vi "Write Size.vi"(8 "error in (no error)":errorcluster, 10 "Coordinate":T1, 11 "Menu in":refnum<class "Menu.lvclass">) -> (0 "error out":errorcluster, 3 "Menu out":refnum<class "Menu.lvclass">)   [LabVIEW 2019, in "RT_Game.lvlib" / "Menu.lvclass"]
uses:
  Menu.lvclass
  Game/Coordinate.ctl
  Menu.lvclass/Menu.ctl
  Game/Game.lvclass
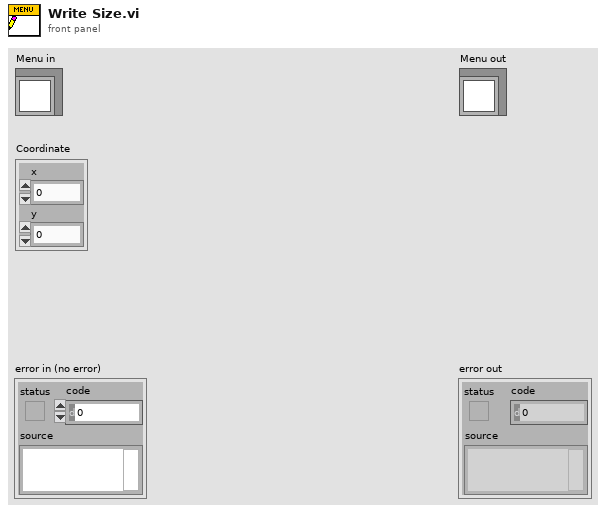
[diagram p1: front panel]
types:
  T1 = typedef "RT_Game.lvlib/Game.lvclass/Coordinate.ctl" = cluster{"x":i16, "y":i16}
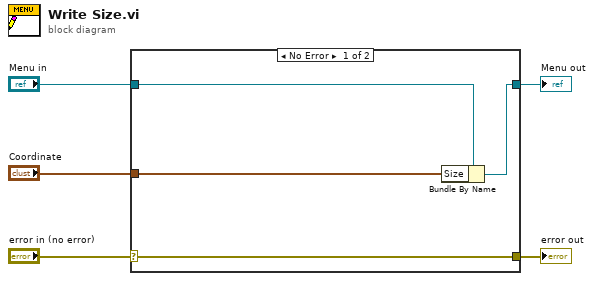
[diagram p0: block diagram]
diagram:
  n1 = case shown="No Error" "error in (no error)" {
    selector: "error in (no error)" -> [w9 w10]
    tunnel: [w9 w10] -> w4
    tunnel: [w7 w11] -> w2
    tunnel: "Menu in" -> [w8 w11]
    tunnel: "Coordinate" -> [w6 _]
    frame No Error {
      n2 = Bundle By Name(cluster=w8, "Size"=w6) -> (w7:refnum<class "Menu.lvclass">)
    }
    frame Error {
    }
  }
  "error out" <- w4
  "Menu out" <- w2
